vi "ContinousLoopMain.vi"(11 "error in":errorcluster) -> (2 "Output Directory":path, 3 "File Prefix":string, 4 "Total Duration":dbl format="%<%H:%M:%S>t", 6 "Interval":dbl format="%<%H:%M:%S>t", 10 "Microscope":T1(array[cluster]), 12 "ProgramStopped":bool, 13 "StartProgram":bool, 14 "Positions":dbl[][](array[numeric]), 15 "error out":errorcluster)   [LabVIEW 2018, in "ContinousLoop.lvlib"]
uses:
  ContinousLoop.lvlib
  Config/Config.lvlib
panel:
  in  "Load file":bool
  in  "Start Program":bool
  in  "stop":bool
  in  "Configuration File":path
  out "Continuous Program":string[][](array[string])
  # "Microscope"
  # "Program Control"
  # "Positions"
  # "Steps"
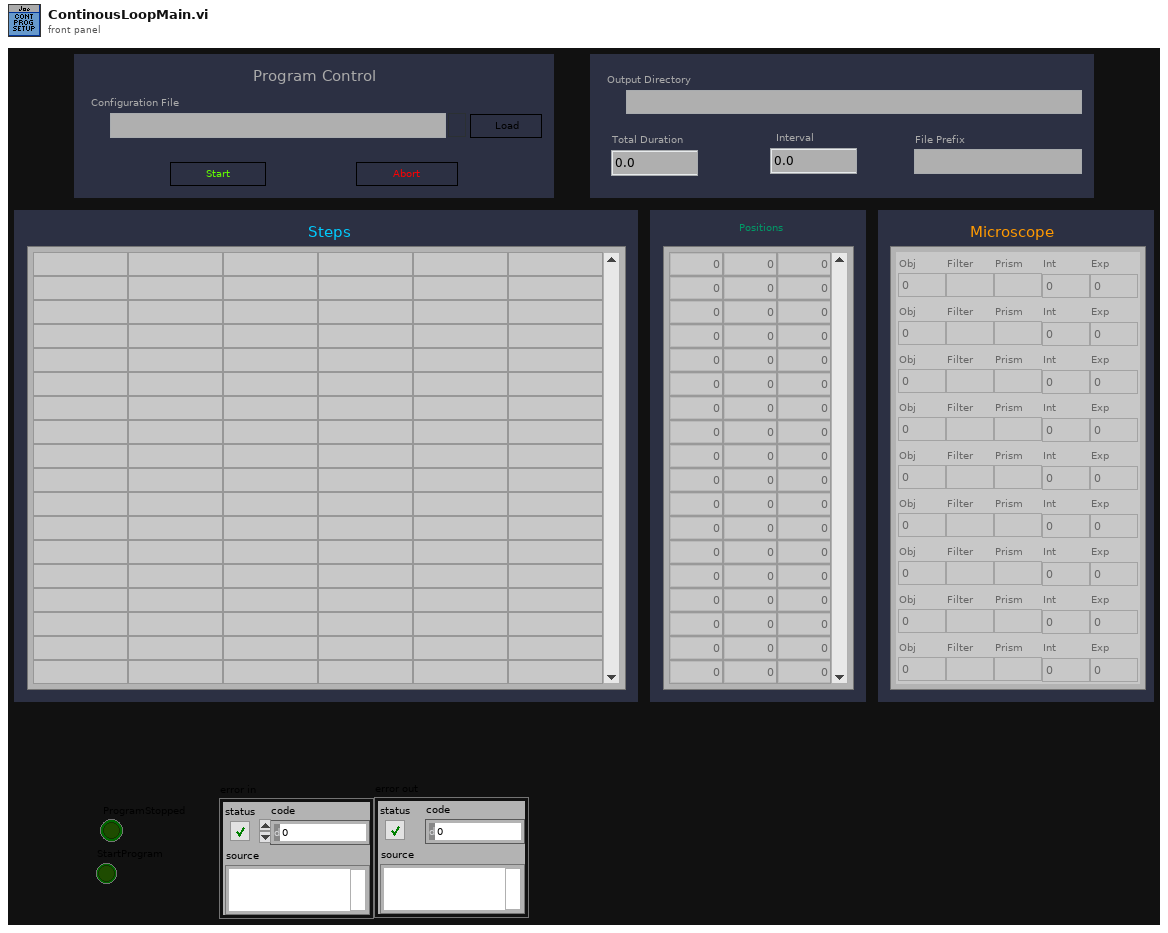
[diagram p1: front panel]
types:
  T1 = cluster{"Obj":i32, "Filter":string, "Prism":string, "Int":dbl, "Exp":i32}[]
  T2 = enum8{"Enabled", "Disabled", "Disabled and Grayed Out"}
  T3 = cluster{"Objective":i32, "Filter":string, "Prism":string, "Intensity":dbl, "Exposure":i32}[]
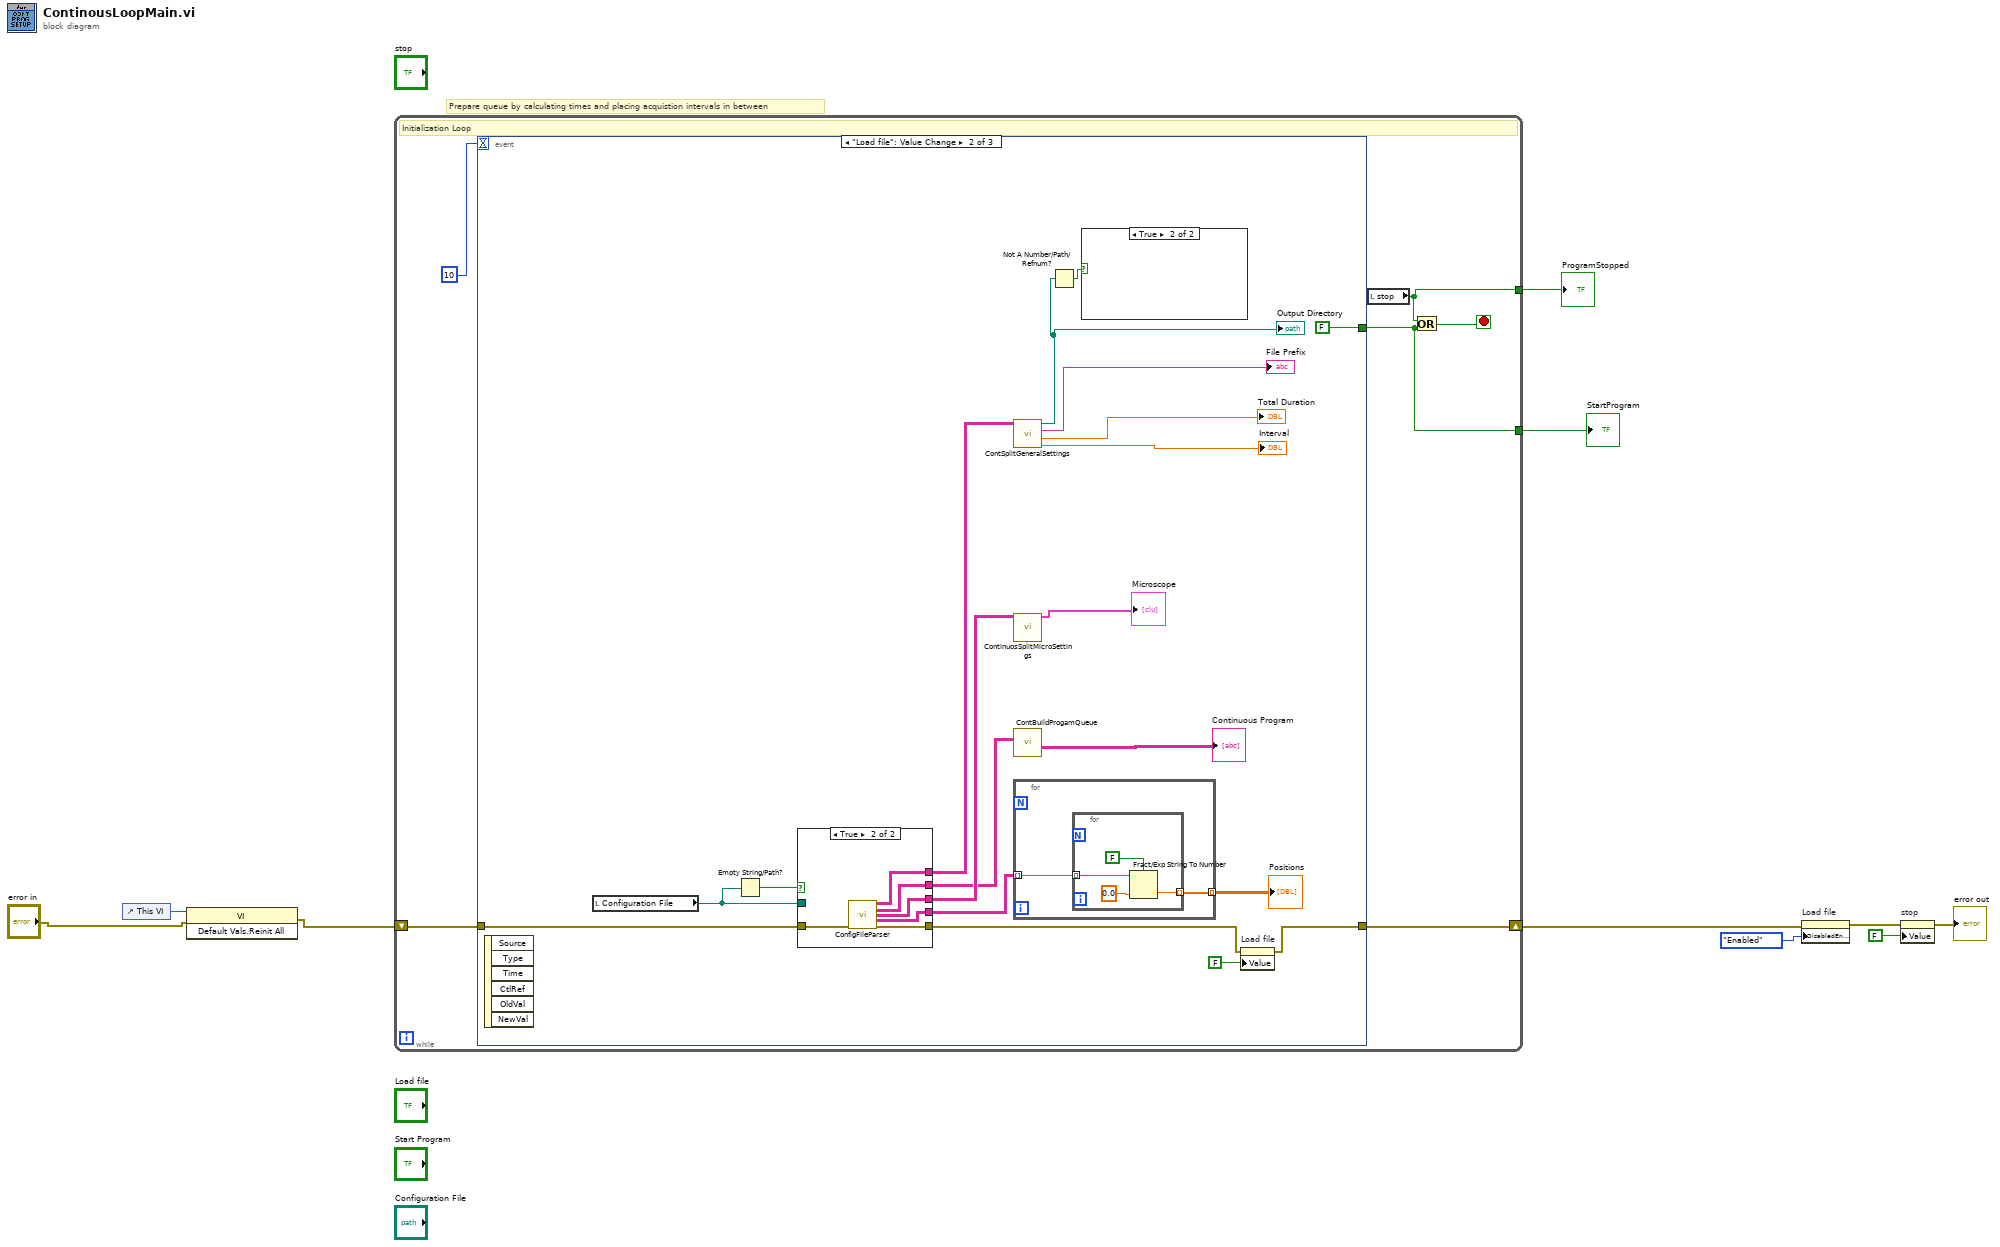
[diagram p0: block diagram]
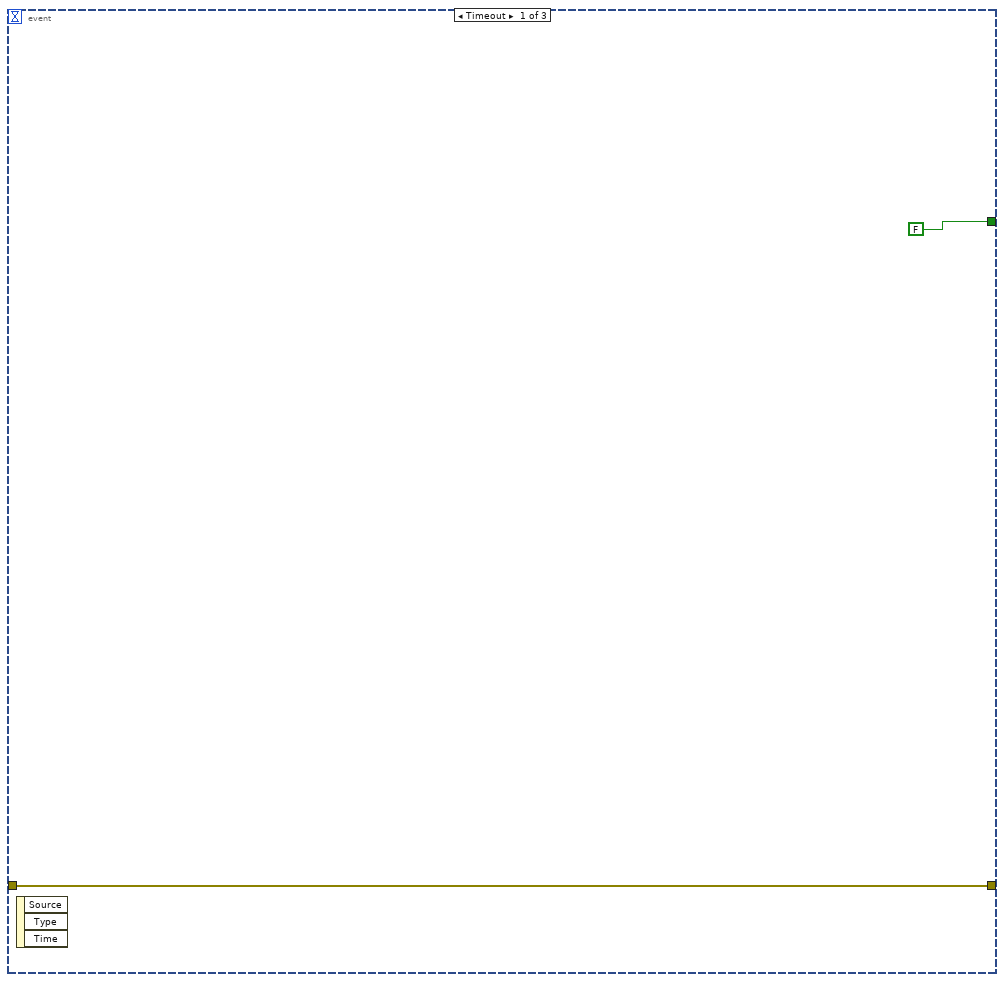
[diagram p2: hidden frame]
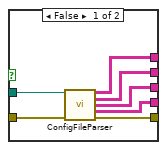
[diagram p4: hidden frame]
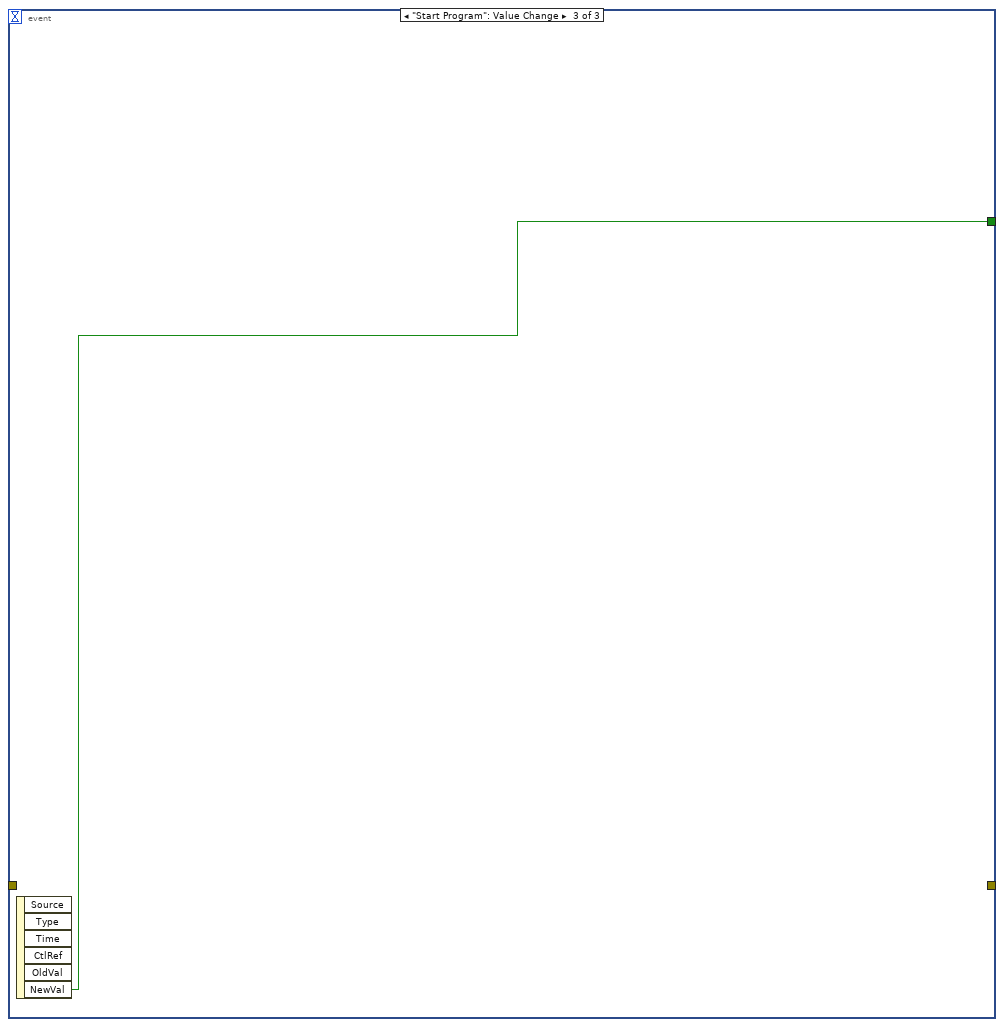
[diagram p5: hidden frame]
diagram:
  # "Prepare queue by calculating times and placing acquistion intervals in between"
  n1 = control-ref of="This VI"() -> (w4:refnum<vi>)
  n2 = invoke class="VI" method="Default Vals.Reinit All"(reference=w4, error in="error in") -> (error out=w3:errorcluster)  [unwired: 1 in, 2 out]
  n3 = while {
    shift-right: [w15] -> w5
    shift-left: w3 -> [w14]
    tunnel: [w12] -> w6
    tunnel: [w11] -> w1
    stop <- w13 stop-if-true
    # "Initialization Loop"
    n4 = event shown="[1] \"Load file\": Value Change" {
      selector: _ -> [_ _ _]
      dyn-events: _ -> [_ _ _]
      timeout: 10 -> [_ _ _]
      tunnel: [w18 w26 _] -> w15
      tunnel: w14 -> [w18 w28 _]
      tunnel: [FALSE ("NewVal") FALSE ("NewVal") w57] -> w12
      event Timeout {
        n5 = event-data() -> ()  [unwired: 1 in, 3 out]
      }
      event "Load file": Value Change {
        n6 = event-data() -> ()  [unwired: 1 in, 6 out]
        n7 = local read "Configuration File"() -> (w34:path)
        n8 = Empty String/Path?(string/path=w34) -> (empty?=w35:bool)
        n9 = case shown="True" w35 {
          tunnel: w34 -> [w50 _]
          tunnel: [w49 w56] -> w29
          tunnel: [w48 w54] -> w36
          tunnel: [w47 w55] -> w32
          tunnel: [w46 w53] -> w31
          tunnel: [w45 w52] -> w25
          tunnel: w28 -> [w44 w51]
          frame False {
            n10 = call "ConfigFileParser.vi"("Path"=w50, "error in"=w44) -> ("General Settings"=w46:string[][], "Program"=w49:string[][], "Loop Microscope Settings"=w47:string[][], "Positions"=w48:string[][], "error out"=w45:errorcluster)  [unwired: 8 in, 1 out]
          }
          frame True {
            n11 = call "ConfigFileParser.vi"("error in"=w51) -> ("General Settings"=w53:string[][], "Program"=w56:string[][], "Loop Microscope Settings"=w55:string[][], "Positions"=w54:string[][], "error out"=w52:errorcluster)  [unwired: 9 in, 1 out]
          }
        }
        n12 = call "ContSplitGeneralSettings.vi"("General Settings"=w31) -> ("Interval"=→"Interval":dbl, "Total Duration"=→"Total Duration":dbl, "File Prefix"=→"File Prefix":string, "SaveDir"=w22:path)  [unwired: 7 in]
        "Output Directory" <- w22
        n13 = call "ContinuosSplitMicroSettings.vi"("Loop Microscope Settings"=w32) -> ("Microscope"=→"Microscope":T3)  [unwired: 14 in]
        n14 = call "ContBuildProgamQueue.vi"("Continuous Program"=w29) -> ("Continuous Program modified"=→"Continuous Program":string[][])  [unwired: 10 in]
        n15 = for {
          tunnel: w36 -> [w39] mode=indexing
          tunnel: [w38] -> w37 mode=indexing
          n16 = for {
            tunnel: w39 -> [w43] mode=indexing
            tunnel: [w42] -> w38 mode=indexing
            n17 = Fract/Exp String To Number(use system decimal point (T)=FALSE, string=w43, default (0 dbl)=0.0 ("default (0 DBL)")) -> (number=w42:dbl)  [unwired: 1 in, 1 out]
          }
        }
        "Positions" <- w37
        n18 = Not A Number/Path/Refnum?(number/path/refnum=w22) -> (NaN/Path/Refnum?=w23:bool)
        n19 = case shown="True" w23 {
          frame False {
          }
          frame True {
          }
        }
        n20 = property on="Load file" class="Bool (strict)"(error in=w25, "Value"=FALSE ("Load file")) -> (error out=w26:errorcluster)  [unwired: 1 in, 1 out]
      }
      event "Start Program": Value Change {
        n21 = event-data() -> ("NewVal"=w57:bool)  [unwired: 1 in, 5 out]
      }
    }
    n22 = local read "stop"() -> (w11:bool)
    n23 = Or(x=w11, y=w12) -> (x .or. y?=w13:bool)
  }
  "StartProgram" <- w6
  "ProgramStopped" <- w1
  n24 = property on="Load file" class="Bool (strict)"(error in=w5, "DisabledEnum"=T2."Enabled" ("Disabled")) -> (error out=w8:errorcluster)  [unwired: 1 in, 1 out]
  n25 = property on="stop" class="Bool (strict)"(error in=w8, "Value"=FALSE ("stop")) -> (error out=→"error out":errorcluster)  [unwired: 1 in, 1 out]
